vi "Model - Get DB Records Array.vi"(8 "error in (no error)":errorcluster, 11 "View Model":T2) -> (0 "error out":errorcluster, 2 "DB Records Array":T1[](array[typedef]), 3 "View Model":T2)   [LabVIEW 2017]
doc: "Get actual value of DB Records Array from DVR"
uses:
  Controls/View Model.ctl
  Controls/Shared Model.ctl
  Error Handler/Controls/Error Model.ctl
  Error Handler/Controls/Error Message.ctl
  Error Handler/Controls/Error Type.ctl
  Configuration/Controls/Config Model.ctl
  Configuration/Controls/Config DB Message.ctl
  Configuration/Controls/Config DB Command.ctl
  Configuration/Controls/Config DB Overhead.ctl
  Configuration/Controls/Config DB Record.ctl
  Controller/Controls/Controller Model.ctl
  Views/Vehicle Position Simulation/Controls/Position.ctl
  Controller/Controls/Controller Overhead.ctl
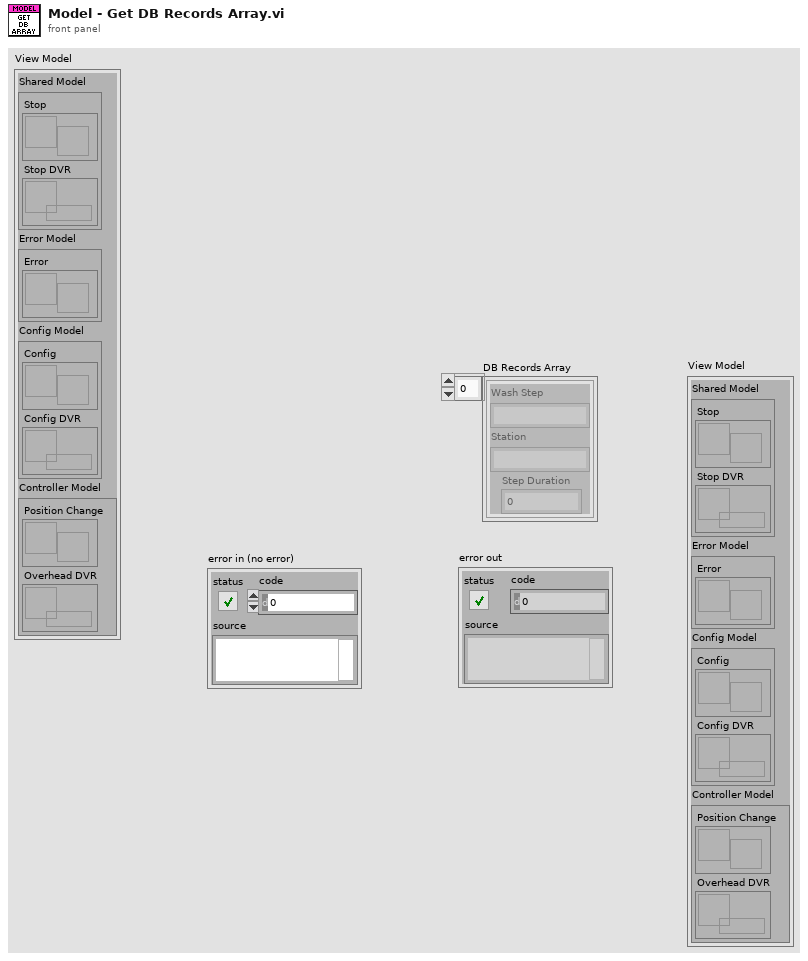
[diagram p1: front panel]
types:
  T1 = typedef "Config DB Record.ctl" = cluster{"Wash Step":string, "Station":string, "Step Duration":u32}
  T2 = typedef "View Model.ctl" = cluster{"Shared Model":T3, "Error Model":T4, "Config Model":T5, "Controller Model":T6}
  T3 = typedef "Shared Model.ctl" = cluster{"Stop":refnum<user-event>, "Stop DVR":refnum<data-value>}
  T4 = typedef "Error Model.ctl" = cluster{"Error":refnum<user-event>}
  T5 = typedef "Config Model.ctl" = cluster{"Config":refnum<user-event>, "Config DVR":refnum<data-value>}
  T6 = typedef "Controller Model.ctl" = cluster{"Position Change":refnum<user-event>, "Overhead DVR":refnum<data-value>}
  T7 = typedef "Config DB Overhead.ctl" = cluster{"Locked DB?":bool, "DB Records Array":T1[], "Queried Step Duration":u32}
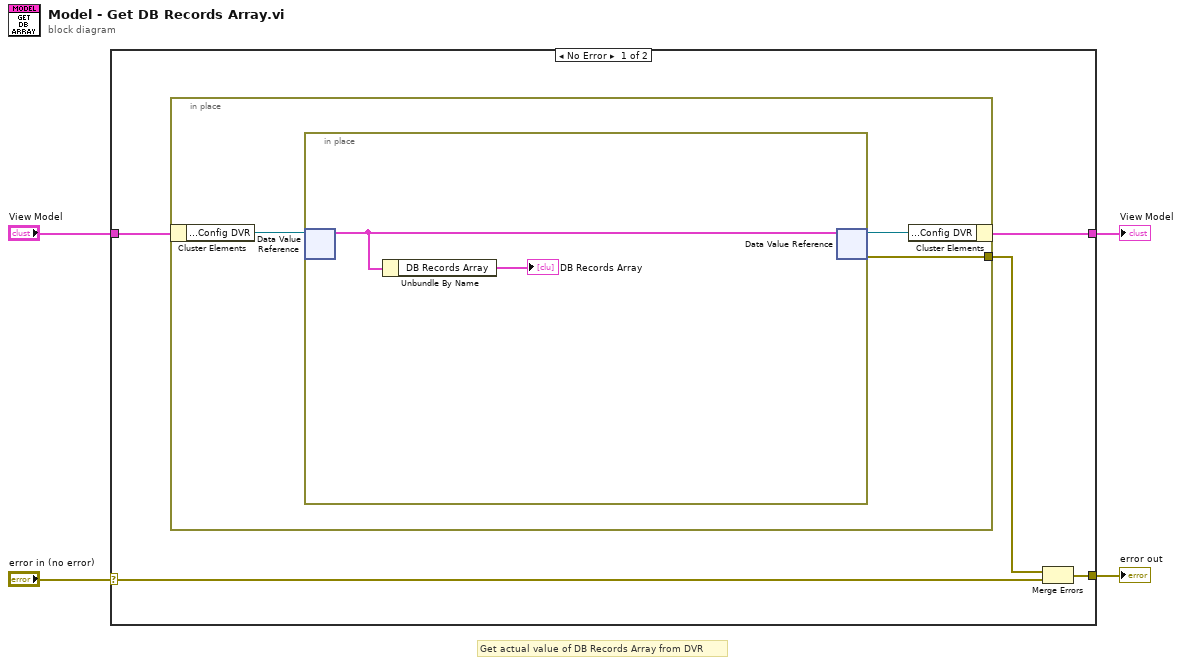
[diagram p0: block diagram]
diagram:
  # "Get actual value of DB Records Array from DVR"
  n1 = case shown="No Error" "error in (no error)" {
    selector: "error in (no error)" -> [w7 w16]
    tunnel: "View Model" -> [w9 w15]
    tunnel: [w6 w16] -> w2
    tunnel: [w5 w15] -> w1
    frame No Error {
      n2 = in-place {
        in-place-border: [w10] -> w8
        n3 = in-place-cluster #1(w9) -> ("Config Model.Config DVR"=w12:refnum<data-value>)
        n4 = in-place {
          n5 = in-place-dvr #2(w12) -> (w14:T7)  [unwired: 1 out]
          n6 = Unbundle By Name(w14) -> ("DB Records Array"=→"DB Records Array":T1[])
          n7 = in-place-dvr #2(w14) -> (w11:refnum<data-value>, w10:errorcluster)
        }
        n8 = in-place-cluster #1("Config Model.Config DVR"=w11) -> (w5:T2)
      }
      n9 = Merge Errors(w8, w7) -> (w6:errorcluster)
    }
    frame Error {
    }
  }
  "View Model" <- w1
  "error out" <- w2
